vi "Task Start.vi"(8 "error in (no error)":errorcluster, 11 "AbortManager in":refnum<class "AbortManager.lvclass">) -> (0 "error out":errorcluster, 3 "AbortManager out":refnum<class "AbortManager.lvclass">)   [LabVIEW 2020, in "Volatus.lvlib" / "AbortManager.lvclass"]
uses:
  AbortManager.lvclass
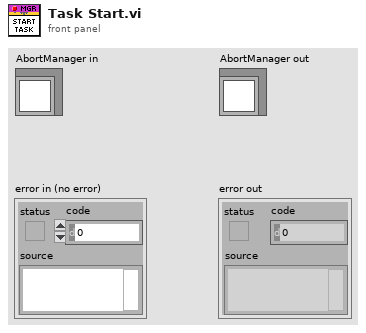
[diagram p1: front panel]
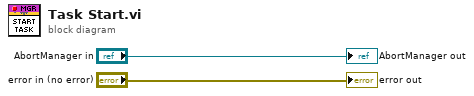
[diagram p0: block diagram]
diagram:
  "error out" <- "error in (no error)"
  "AbortManager out" <- "AbortManager in"
